vi "discover class type.vi"(8 "error in":errorcluster, 10 "class cache data in":T1, 11 "Path":path) -> (0 "error out":errorcluster, 2 "class cache data out":T1)   [LabVIEW 2013, in "PL_class cache.lvlib"]
uses:
  PL_class cache.lvlib
  cached class information.ctl
  target class metadata.ctl
  class metadata.ctl
  <vilib>/NI/Tag Bus Module Framework/root configuration/Target Types.ctl
  <vilib>/NI/Tag Bus Module Framework/root configuration/TBM configuration.lvclass
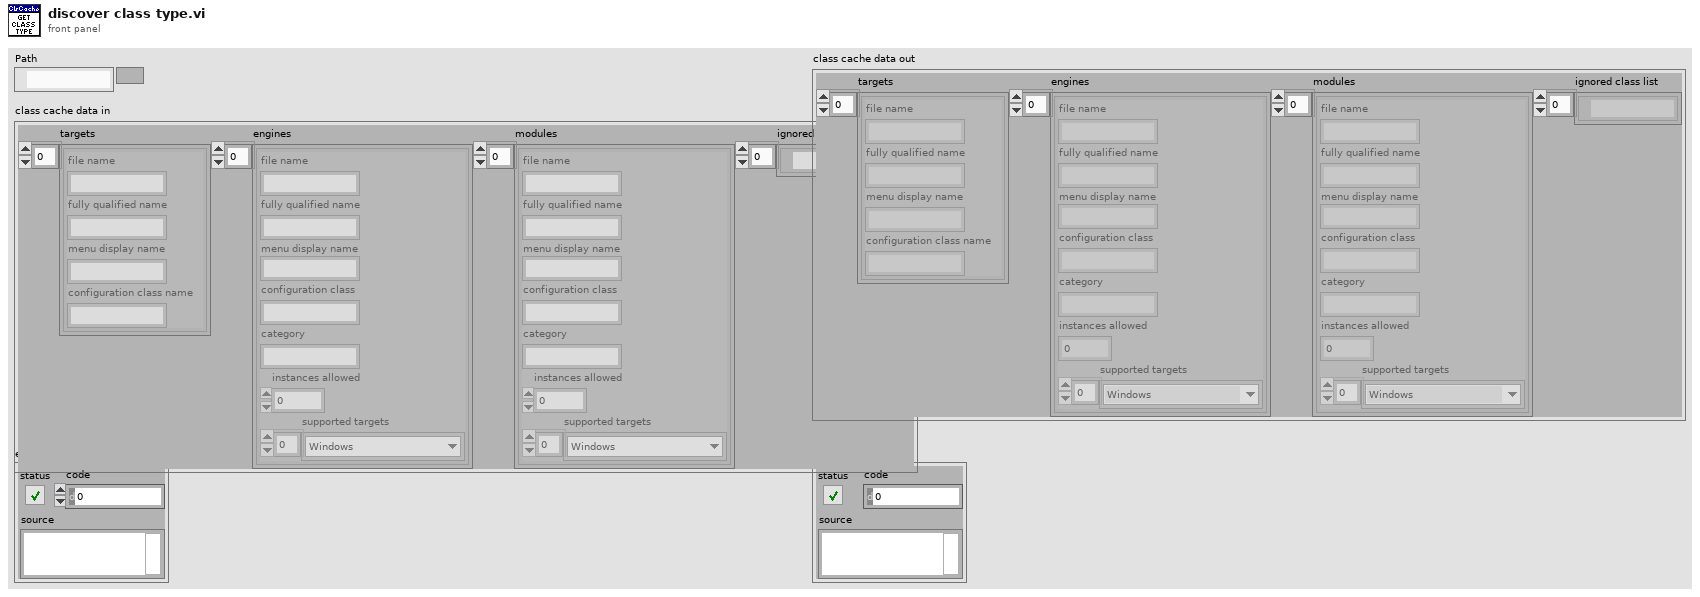
[diagram p1: front panel]
types:
  T1 = typedef "PL_class cache.lvlib/cached class information.ctl" = cluster{"targets":T2[], "engines":T3[], "modules":T3[], "ignored class list":path[]}
  T2 = typedef "PL_class cache.lvlib/target class metadata.ctl" = cluster{"file name":string, "fully qualified name":string, "menu display name":string, "configuration class name":string}
  T3 = typedef "PL_class cache.lvlib/class metadata.ctl" = cluster{"file name":string, "fully qualified name":string, "menu display name":string, "configuration class":string, "category":string, "instances allowed":i32, "supported targets":T4[]}
  T4 = typedef "TBM configuration.lvclass/Target Types.ctl" = enum16{"Windows", "Mac", "Linux", "Linux RT ARM", "VxWorks", "Pharlap", "Other", "Linux RT x64"}
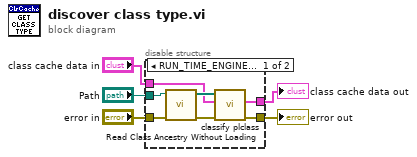
[diagram p0: block diagram]
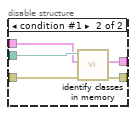
[diagram p2: hidden frame]
diagram:
  n1 = disable-structure shown="RUN_TIME_ENGINE==False" {
    disable-tunnel: [w12 w15] -> w5
    disable-tunnel: "Path" -> [w11 w16]
    disable-tunnel: "error in" -> [w8 w17]
    disable-tunnel: "class cache data in" -> [w7 w14]
    disable-tunnel: [w6 w13] -> w1
    frame condition #0 (active) {
      n2 = call "Read Class Ancestry Without Loading.vi"("error in"=w8, "LabVIEW Class Path"=w11) -> ("error out"=w10:errorcluster, "Class Ancestry"=w9:path[])  [unwired: 8 in]
      n3 = call "classify plclass.vi"("error in"=w10, "class cache data in"=w7, "Class Ancestry"=w9) -> ("error out"=w12:errorcluster, "class cache data out"=w6:T1)  [unwired: 7 in]
    }
    frame condition #1 {
      n4 = call "identify classes in memory.vi"("error in"=w17, "class cache data in"=w14, "Path"=w16) -> ("error out"=w15:errorcluster, "class cache data out"=w13:T1)  [unwired: 7 in]
    }
  }
  "error out" <- w5
  "class cache data out" <- w1
